vi "LHF.DB.Mongo.Database.GetCollection.vi"(0 "LHF.DB.Mongo in":refnum<class "LHF.DB.Mongo.lvclass">, 1 "collectionName":string, 5 "error in (no error)":errorcluster) -> (14 "LHF.DB.Mongo in":refnum<class "LHF.DB.Mongo.lvclass">, 15 "MongoCollection":refnum<k24>, 19 "error out":errorcluster)   [LabVIEW 2013, in "LHF.DB.Mongo.lvclass"]
uses:
  LHF.DB.Mongo.lvclass
  C:/Users/schim/Desktop/Projetos/LabVIEW-MongoDB/src/Driver/MongoDB.Driver.dll
  Driver/MongoDB.Driver.dll
  LHF.DB.Mongo.lvclass/LHF.DB.Mongo.ctl
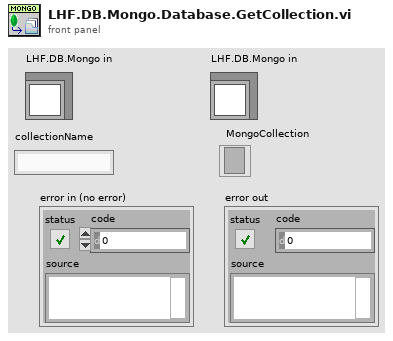
[diagram p1: front panel]
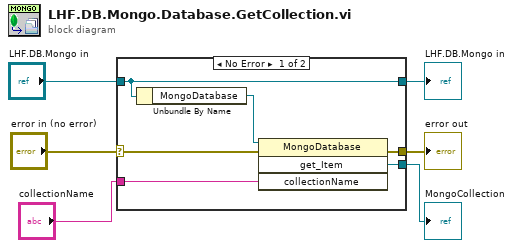
[diagram p0: block diagram]
diagram:
  n1 = case shown="No Error" "error in (no error)" {
    selector: "error in (no error)" -> [w8 w13]
    tunnel: [w12 w13] -> w6
    tunnel: [w11 _] -> w5
    tunnel: "collectionName" -> [w10 _]
    tunnel: "LHF.DB.Mongo in" -> [w7 w14]
    tunnel: [w7 w14] -> w1
    frame No Error {
      n2 = Unbundle By Name(w7) -> ("MongoDatabase"=w9:refnum<k24>)
      n3 = invoke class="MongoDatabase" method="get_Item"(reference=w9, error in=w8, "collectionName"=w10) -> (error out=w12:errorcluster, "get_Item"=w11:refnum<k24>)  [unwired: 1 in, 2 out]
    }
    frame Error {
    }
  }
  "error out" <- w6
  "LHF.DB.Mongo in" <- w1
  "MongoCollection" <- w5
